vi "例4-16.vi"() -> ()   [LabVIEW 2019]
panel:
  in  "学生簇":T1={"学号"=201904012, "姓名"="李大山", "性别"="男", "年龄"=18.0}
  out "年龄":dbl=18.0
  out "性别":string="男"
  out "姓名":string="李大山"
  out "学号":u32=201904012
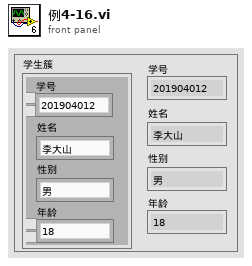
[diagram p1: front panel]
types:
  T1 = cluster{"学号":u32, "姓名":string, "性别":string, "年龄":dbl}
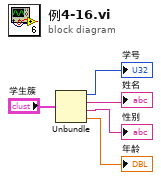
[diagram p0: block diagram]
diagram:
  n1 = Unbundle("学生簇") -> ("学号"=→"学号":u32, "姓名"=→"姓名":string, "性别"=→"性别":string, "年龄"=→"年龄":dbl)
